vi "Sweep Mode (Set).vi"(6 "ISOBUS address":T2=-1 caption="ISOBUS address (-1)", 8 "error in":errorcluster, 10 "Sweep Mode":string, 11 "Mercury Reference In":T4) -> (0 "error out":errorcluster, 2 "Response":T1, 3 "Mercury Reference Out":T4, 4 "Valid?":T3)   [LabVIEW 2013, in "Mercury iXX.lvlib" / "Control Loop.lvlib"]
doc: "Set the sweep mode."
uses:
  Control Loop.lvlib
  Mercury iXX.lvlib
  Private/Controls/Command Verbs.ctl
  Controls/Response String.ctl
  Controls/Is Valid LED.ctl
  Controls/Comms Transport Layer.ctl
  Private/Controls/Query Dynamic Reference.ctl
  Controls/Mercury Reference.ctl
  Controls/ISOBus Address.ctl
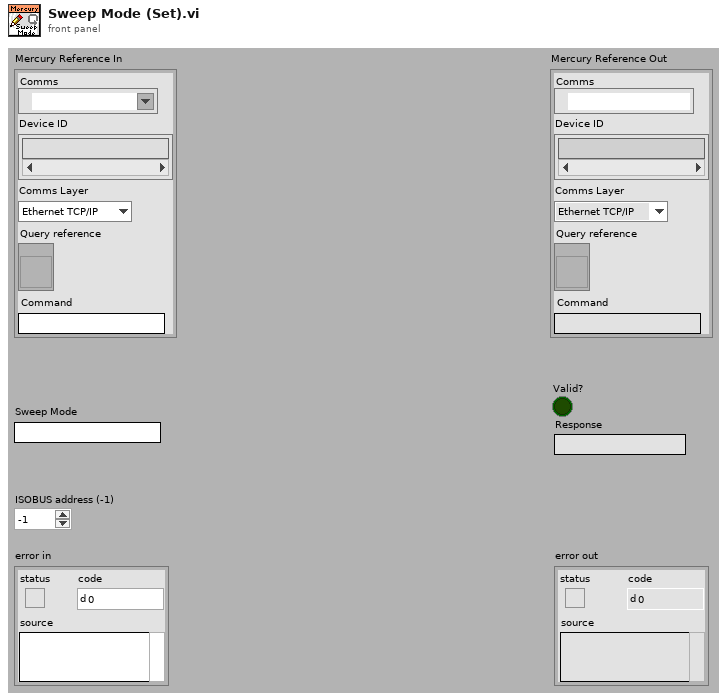
[diagram p1: front panel]
types:
  T1 = typedef "Mercury iXX.lvlib/Response String.ctl" = string
  T2 = typedef "Mercury iXX.lvlib/ISOBus Address.ctl" = i32
  T3 = typedef "Mercury iXX.lvlib/Is Valid LED.ctl" = bool
  T4 = typedef "Mercury iXX.lvlib/Mercury Reference.ctl" = cluster{"Comms":refnum<visa-resource-name>, "Device ID":string[], "Comms Layer":T5, "Command":string, "Query reference":T6}
  T5 = typedef "Mercury iXX.lvlib/Comms Transport Layer.ctl" = enum16{"Ethernet TCP/IP", "USB", "ISOBus - RS-232", "GPIB"}
  T6 = typedef "Mercury iXX.lvlib/Query Dynamic Reference.ctl" = refnum<vi>
  T7 = typedef "Mercury iXX.lvlib/Command Verbs.ctl" = string
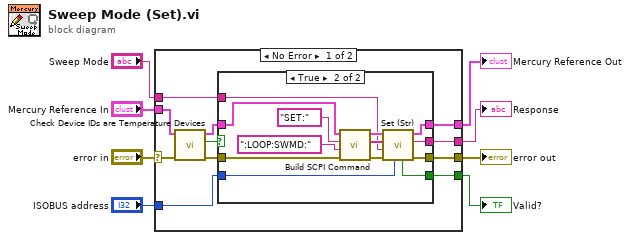
[diagram p0: block diagram]
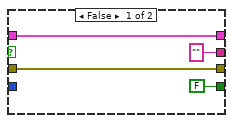
[diagram p2: hidden frame]
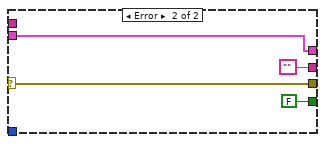
[diagram p3: hidden frame]
diagram:
  n1 = case shown="No Error" "error in" {
    selector: "error in" -> [w14 w39]
    tunnel: "Mercury Reference In" -> [w12 w40]
    tunnel: [w17 w40] -> w7
    tunnel: [w16 w39] -> w1
    tunnel: "ISOBUS address" -> [w18 _]
    tunnel: [w10 ""] -> w3
    tunnel: [w9 FALSE ("Valid?")] -> w2
    tunnel: "Sweep Mode" -> [w19 _]
    frame No Error {
      n2 = call "Check Device IDs are Temperature Devices.vi"("error in"=w14, "Mercury Reference In"=w12) -> ("error out"=w13:errorcluster, "Valid?"=w15:bool, "Mercury Reference Out"=w11:T4)  [unwired: 7 out]
      n3 = case shown="True" w15 {
        tunnel: w19 -> [_ w26]
        tunnel: w13 -> [w23 w27]
        tunnel: w18 -> [_ w24]
        tunnel: w11 -> [w22 w31]
        tunnel: [w22 w32] -> w17
        tunnel: [w23 w30] -> w16
        tunnel: [T1 "" ("Response") w29] -> w10
        tunnel: [T3 FALSE ("Valid?") w28] -> w9
        frame False {
        }
        frame True {
          n4 = call "Build SCPI Command.vi"("error in"=w27, "Noun(s)"=":LOOP:SWMD:" ("Command"), "Verb"=T7 "SET:", "Mercury Reference In"=w31) -> ("error out"=w33:errorcluster, "SCPI Message(s)"=w34:string[], "Mercury Reference Out"=w35:T4)  [unwired: 5 out]
          n5 = call "Set (Str).vi"("ISOBUS address"=w24, "error in"=w33, "Command Value (Str)"=w26, "SCPI Message(s)"=w34, "Mercury Reference In"=w35) -> ("error out"=w30:errorcluster, "Response"=w29:T1, "Mercury Reference Out"=w32:T4, "Valid?"=w28:T3)  [unwired: 3 out]
        }
      }
    }
    frame Error {
    }
  }
  "Mercury Reference Out" <- w7
  "error out" <- w1
  "Valid?" <- w2
  "Response" <- w3
